vi "python.vi"(11 "Image Pixels (U32)":u32[][](array[numeric])) -> (0 "error out":errorcluster, 3 "Array":u32[][](array[numeric]))   [LabVIEW 2020]
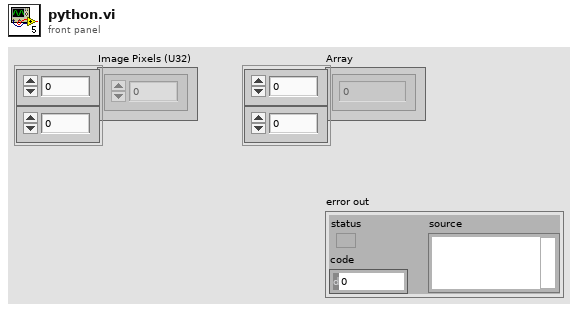
[diagram p1: front panel]
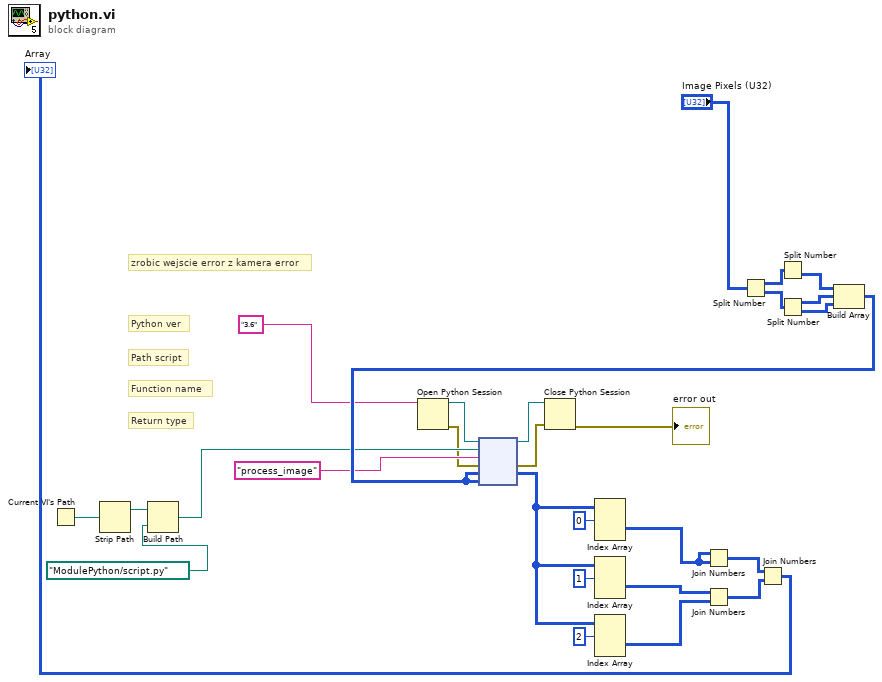
[diagram p0: block diagram]
diagram:
  # "Function name"
  # "zrobic wejscie error z kamera error"
  # "Python ver"
  # "Path script"
  # "Return type"
  n1 = Current VI's Path() -> (path=w8:path)
  n2 = Strip Path(path=w8) -> (stripped path=w9:path)  [unwired: 1 out]
  n3 = Build Path(base path=w9, name or relative path=path "ModulePython/script.py" ("module path")) -> (appended path=w11:path)
  n4 = Open Python Session(python version="3.6") -> (session out=w1:refnum<k35>, error out=w4:errorcluster)  [unwired: 2 in]
  n5 = Split Number(x="Image Pixels (U32)") -> (hi(x)=w12:u16[][], lo(x)=w13:u16[][])
  n6 = Split Number(x=w12) -> (lo(x)=w17:u8[][])  [unwired: 1 out]
  n7 = Split Number(x=w13) -> (hi(x)=w16:u8[][], lo(x)=w15:u8[][])
  n8 = Build Array(w17, w16, w15) -> (w18:u8[][][])
  n9 = node(w1, w11, "process_image" ("function name"), w4, w18, w18) -> (w2:refnum<k35>, w5:errorcluster, w19:u8[][][])  [unwired: 1 in, 2 out]
  n10 = Close Python Session(session in=w2, error in=w5) -> (11:→"error out":errorcluster)
  n11 = Index Array(array=w19, index (dim 0)=0 ("index (page)")) -> (element=w28:u8[][])  [unwired: 2 in]
  n12 = Index Array(array=w19, index (dim 0)=1 ("index (page)")) -> (element=w25:u8[][])  [unwired: 2 in]
  n13 = Index Array(array=w19, index (dim 0)=2 ("index (page)")) -> (element=w26:u8[][])  [unwired: 2 in]
  n14 = Join Numbers(hi=w28, lo=w28) -> ((hi.lo)=w23:u16[][])
  n15 = Join Numbers(hi=w25, lo=w26) -> ((hi.lo)=w24:u16[][])
  n16 = Join Numbers(hi=w23, lo=w24) -> ((hi.lo)=→"Array":u32[][])
